vi "Ack.vi"(0 "STOMP in":refnum<class "STOMP.lvclass">, 2 "ack id":string, 5 "error in (no error)":errorcluster, 6 "Receipt?":bool) -> (14 "STOMP out":refnum<class "STOMP.lvclass">, 19 "error out":errorcluster)   [LabVIEW 2017, in "LabVIEW STOMP.lvlib" / "STOMP.lvclass"]
uses:
  STOMP.lvclass
  Typedefs/Type_ClientFrame.ctl
  Typedefs/Type_ClientFrameType.ctl
  Typedefs/Type_FrameHeader.ctl
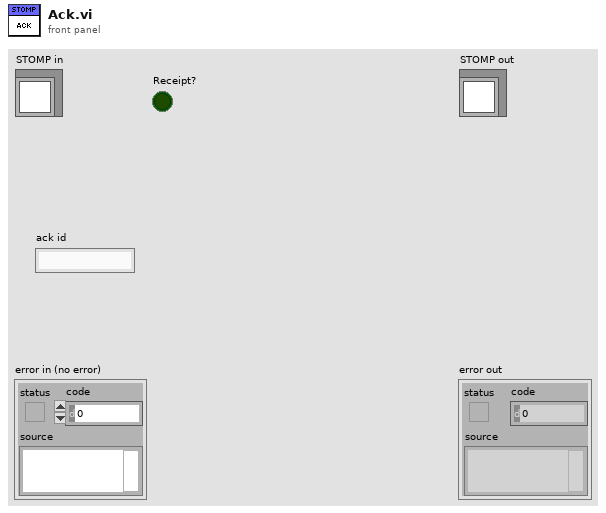
[diagram p1: front panel]
types:
  T1 = typedef "LabVIEW STOMP.lvlib/STOMP.lvclass/Type_FrameHeader.ctl" = cluster{"Header":string, "Value":string}
  T2 = typedef "LabVIEW STOMP.lvlib/STOMP.lvclass/Type_ClientFrameType.ctl" = enum16{"Undefined", "SEND", "SUBSCRIBE", "UNSUBSCRIBE", "BEGIN", "COMMIT", "ABORT", "ACK", "NACK", "DISCONNECT"}
  T3 = typedef "LabVIEW STOMP.lvlib/STOMP.lvclass/Type_ClientFrame.ctl" = cluster{"Type":T2, "Headers":T1[], "Body":string}
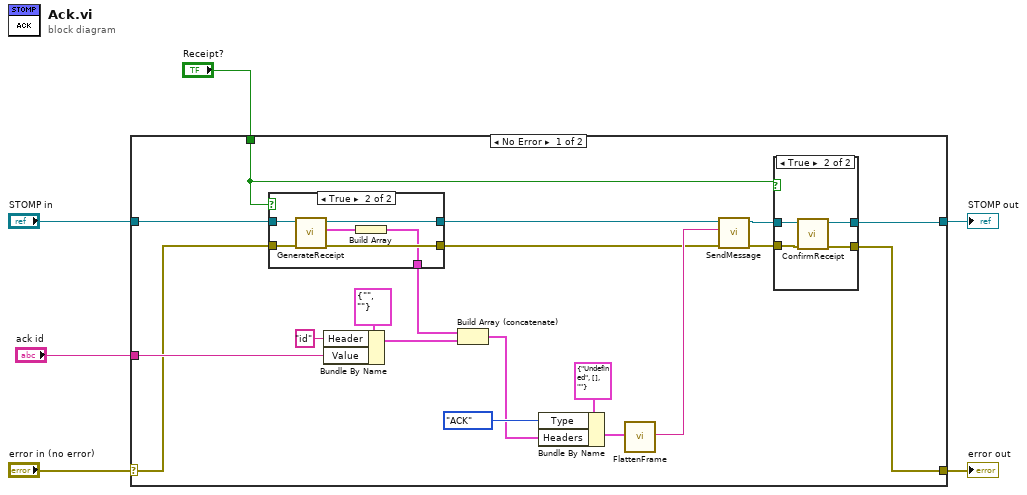
[diagram p0: block diagram]
diagram:
  n1 = case shown="No Error" "error in (no error)" {
    selector: "error in (no error)" -> [w15 w41]
    tunnel: [w9 w41] -> w5
    tunnel: [w8 w40] -> w3
    tunnel: "STOMP in" -> [w16 w40]
    tunnel: "ack id" -> [w23 _]
    tunnel: "Receipt?" -> [w7 _]
    frame No Error {
      n2 = case shown="True" w7 {
        tunnel: w16 -> [w27 w33]
        tunnel: w15 -> [w26 w32]
        tunnel: [w27 w31] -> w14
        tunnel: [w26 w30] -> w13
        tunnel: [_ w28] -> w12
        frame False {
        }
        frame True {
          n3 = call-dynamic "GenerateReceipt.vi"("error in (no error)"=w32, "STOMP in"=w33) -> ("error out"=w30:errorcluster, "Receipt Header"=w29:T1, "STOMP out"=w31:refnum<class "STOMP.lvclass">)  [unwired: 7 in]
          n4 = Build Array(w29) -> (w28:T1[])
        }
      }
      n5 = Bundle By Name(cluster=T1 {"Header"="", "Value"=""}, "Header"="id", "Value"=w23) -> (w21:T1)
      n6 = Build Array (concatenate)(w12, w21) -> (w20:T1[])
      n7 = Bundle By Name(cluster=T3 {"Type"=enum."Undefined", "Headers"=[], "Body"=""} ("Type_ClientFrame"), "Type"=Type_ClientFrameType."ACK", "Headers"=w20) -> (w19:T3)
      n8 = call "FlattenFrame.vi"("Client Frame"=w19) -> ("flattened frame"=w18:string)  [unwired: 18 in]
      n9 = call-dynamic "SendMessage.vi"("error in (no error)"=w13, "data in"=w18, "STOMP in"=w14) -> ("error out"=w10:errorcluster, "STOMP out"=w11:refnum<class "STOMP.lvclass">)  [unwired: 7 in]
      n10 = case shown="True" w7 {
        tunnel: w11 -> [w34 w39]
        tunnel: w10 -> [w35 w38]
        tunnel: [w35 w37] -> w9
        tunnel: [w34 w36] -> w8
        frame False {
        }
        frame True {
          n11 = call-dynamic "ConfirmReceipt.vi"("error in (no error)"=w38, "STOMP in"=w39) -> ("error out"=w37:errorcluster, "STOMP out"=w36:refnum<class "STOMP.lvclass">)  [unwired: 8 in]
        }
      }
    }
    frame Error {
    }
  }
  "error out" <- w5
  "STOMP out" <- w3
